vi "FGV DUT steps.vi"(10 "Enum":enum16{"write", "read"}(ring)=enum."read", 11 "SapID":string) -> (3 "Steps OUT":string[](array[string]))   [LabVIEW 2018]
panel:
  out "text":string
  out "error out":errorcluster
  in  "error in (no error)":errorcluster
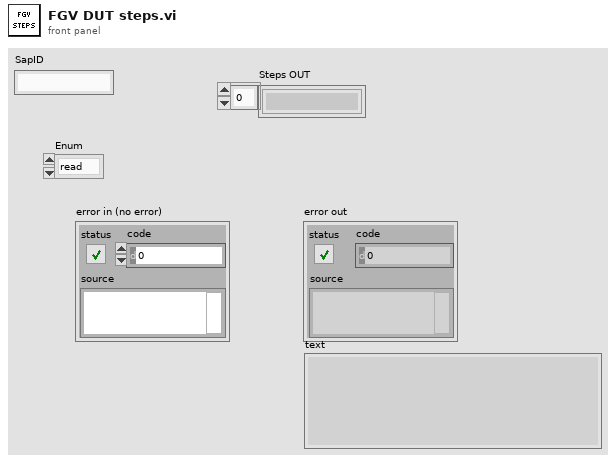
[diagram p1: front panel]
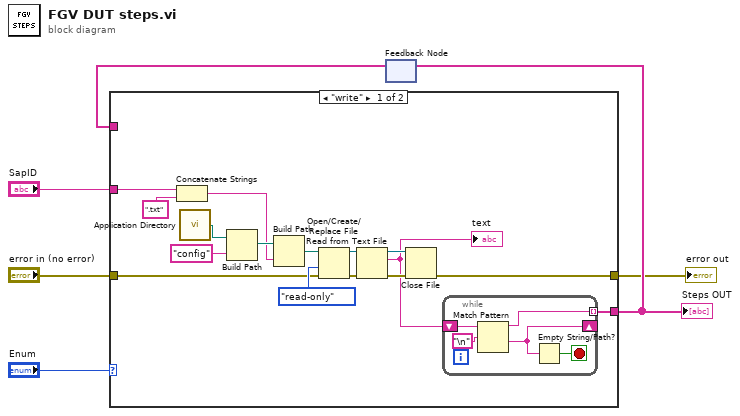
[diagram p0: block diagram]
diagram:
  n1 = feedback #1() -> (w5:string[])  [unwired: 1 in]
  n2 = case shown="\"write\"" "Enum" {
    tunnel: w5 -> [_ w29]
    tunnel: [w7 w29] -> w4
    tunnel: "SapID" -> [w10 _]
    tunnel: "error in (no error)" -> [w9 w28]
    tunnel: [w8 w28] -> w1
    frame "write" {
      n3 = Concatenate Strings(w10, ".txt") -> (w13:string)
      n4 = call <vilib>:"Application Directory.vi"() -> ("Application Directory"=w15:path)
      n5 = Build Path(base path=w15, name or relative path="config") -> (appended path=w14:path)
      n6 = Build Path(base path=w14, name or relative path=w13) -> (appended path=w12:path)
      n7 = Open/Create/Replace File(file path (use dialog)=w12, error in=w9, access (0:read/write)=enum16{"read/write", "read-only", "write-only"}."read-only") -> (refnum out=w20:refnum<file>, error out=w19:errorcluster)  [unwired: 3 in, 1 out]
      n8 = Read from Text File(file (use dialog)=w20, error in=w19) -> (refnum out=w17:refnum<file>, text=w11:string, error out=w18:errorcluster)  [unwired: 2 in, 1 out]
      "text" <- w11
      n9 = Close File(refnum=w17, error in=w18) -> (error out=w8:errorcluster)  [unwired: 1 out]
      n10 = while {
        shift-right: [w24] -> _
        shift-left: w11 -> [w27]
        tunnel: [w25] -> w7 mode=indexing
        stop <- w23 stop-if-true
        n11 = Match Pattern(string=w27, regular expression="\n") -> (before substring=w25:string, after substring=w24:string)  [unwired: 1 in, 2 out]
        n12 = Empty String/Path?(string/path=w24) -> (empty?=w23:bool)
      }
    }
    frame "read", Default {
    }
  }
  "Steps OUT" <- w4
  "error out" <- w1
  n13 = feedback-in #1(w4) -> ()
